vi "Laurel Meter Continuous Gather Tester.vi"(8 "Error In":errorcluster) -> (0 "Error Out":errorcluster)   [LabVIEW 2016]
uses:
  Trunk/Washer DOE/Type Definitions/DOE Test Fixture Hardware.ctl
  Trunk/Utility/Type Definitions/UTILITY Power Inputs Control.ctl
  IND560 Scale Monitor/Type Definitions/IND560 Configuration.ctl
  Trunk/Hybrid Water Heater/Type Definitions/HEWH Agilent Cluster.ctl
  Trunk/Utility/Type Definitions/UTILITY TC Coefficients.ctl
  Omega FMA-1600A Series Gas Flow Meter/Type Definitions/FMA1600A COM Ports.ctl
  Trunk/Washer DOE/Type Definitions/DOE Front Panel Meters.ctl
  Trunk/Utility/Type Definitions/UTILITY Power Data.ctl
  Trunk/Utility/Standby Power/Type Definitions/Standby Power Main Data.ctl
  Omega FMA-1600A Series Gas Flow Meter/Type Definitions/FMA1600A Gas Data.ctl
  Omega FMA-1600A Series Gas Flow Meter/Type Definitions/FMA1600A Gas Type.ctl
  Trunk/Range/Type Definitions/RANGE Meter Selector.ctl
  <vilib>/ptbypt/NI_PtbyPt.lvlib
panel:
  in  "Collect Meter (HOT,COLD,HOT COLD)":string
  in  "Laurel Communication Type":string
  in  "Rinse Button?":bool
  out "Loop Rate":dbl format="%0.2f"
  out "Header Data":string[][](array[string])
  in  "Measurments":T1 {"Power Measurements"."Voltage (V):Element 1 Avg" format="%.3g"; "Power Measurements"."Voltage (V):Element 2 Avg" format="%.3g"; "Power Measurements"."Max Watt Hours" format="%.3g"; "Power Measurements"."Power Factor:Element 2" format="%.3g"; "Power Measurements"."Power Factor:Element 1" format="%.3g"; "Power Measurements"."Apparent Power (VA):Element 2" format="%.3g"; "Power Measurements"."Apparent Power (VA):Element 1" format="%.3g"; "Power Measurements"."Frequency (Hz):Element 1" format="%.3g"; "Power Measurements"."Time:Element 1" format="%.3g"; "Power Measurements"."Voltage Crest Factor:Element 2" format="%.3g"; "Power Measurements"."Voltage Crest Factor:Element 1" format="%.3g"; "Power Measurements"."Voltage Harmonic Content (%):Element 2" format="%.3g"; "Power Measurements"."Voltage Harmonic Content (%):Element 1" format="%.3g"; "Power Measurements"."Current Crest Factor:Element 2" format="%.3g"; "Power Measurements"."Current Crest Factor:Element 1" format="%.3g"; "Power Measurements"."Voltage (V):Element 1" format="%.3g"; "Power Measurements"."Voltage (V):Element 2" format="%.3g"; "Power Measurements"."Watt Hours (Wh):Sigma" format="%.3g"; "Power Measurements"."Power (W):Sigma" format="%.3g"; "Power Measurements"."Current (A):Element 2" format="%.3g"; "Power Measurements"."Current (A):Element 1" format="%.3g"}
  in  "Fixture Hardware":T7={"Power "={"Yokogawa"={"WT210"={"Sample Rate (1: 0.25s)"=1, "A Range (12: 20A)"=11, "V Range (6: 600V)"=4, "Power VISA Yokogawa WT210"=""}, "WT500"={"Power VISA Yokogawa WT500"="", "V Range (8: 1000V)"=6, "I Range (7: 40A)"=7, "Update Rate (3: 500ms)"=2}, "WT310_2"={"Sample Rate (1: 0.25s)"=1, "A Range (12: 20A)"=11, "V Range (6: 600V)"=4, "Power VISA Yokogawa WT310_2"="WT310_2"}, "WT310_3"={"Sample Rate (1: 0.25s)"=1, "A Range (12: 20A)"=11, "V Range (6: 600V)"=4, "Power VISA Yokogawa WT310_3"="WT310_3"}}, "Aplus"={"Aplus IP Address"="192.168.1.101", "Remote Port"=502, "Instrument"="APLUS", "Instr Driver Revision"="1.03.0053"}, "Power Limits"={"Crest Factor"={"Upper Limit"=1.49, "Lower Limit"=1.34}, "Harmonic Content"={"Uthd"=2.0}, "Voltage"={"% Error"=2.0}, "Stability"={"<1 Watt "={"Wattage"=1.0, "Slope (mW/H)"=10.0}, ">1 Watt"={"1%Power/Hour"=1.0}}}, "Nominal Voltage"=120, "Time Limit (s)"=10800.0, "Power Variation Limit (%)"=50.0, "Power Supply"={"Chroma 61605"="CHROMA", "Use Chroma?"=FALSE}}, "Weight Scale"={"Com Options"={"IND560Scale VISA"="MW100", "IP Address"="", "Remote Port"=502, "Setra Scale VISA"="SETRA", "GSE 350"="GSE350"}, "Select Scale"=""}, "Flow Rates"={"Laurel Cold IP Address"="10.0.3.4", "Laurel Hot IP Address"="10.0.3.3", "Hot Water Laurel VISA"="LaurelMeter_Hot", "Cold Water Laurel VISA"="LaurelMeter_Cold", "Remote Port"=0, "Laurel Communication Type"="", "Meters To Collect (Hot Cold)"="", "HOT Laurel Reference"=refnum, "COLD Laurel Reference"=refnum}, "Analog Data"={"Agilent"={"Agilent 34972_1"="34972A_1", "Agilent 34972_2"="34972A_2", "Agilent 34972_3"="34972A_3", "Agilent 34972_4"="34972A_3", "Agilent 34972_5"="34972A_3", "Agilent 34972_6"="34972A_3", "Agilent Gain"=0.0, "TC Type (K,J,T)"="", "Instrument IDN?"="", "TC Channels-List"="", "Analog Channels-List"="", "Agilent Cluster Array"=[], "TC Channels-List 2"="", "Analog Channels-List 2"=""}, "Yokogawa"={"MW100"="MW100", "Intellifaucet"=FALSE}, "Select Analog"="", "TC Coefficients"={"TC Coefficients 1"=[], "TC Coefficients 2"=[], "TC Coefficients 3"=[], "TC Coefficients 4"=[], "TC Coefficients 5"=[], "TC Coefficients 6"=[], "TC Coefficients 7"=[]}, "NI Tasks (Dryer DOE)"=["TC Temps-Module 1", "TC Temps-Module 2", "TC Temps-Module 3", "TC Temps-Module 4", "TC Temps-Module 5", "Gas and Temp-Module 6", "AC_DC Events-Module 7"], "Laurel Analog"={"Laurel IP (Water Temp)"="", "Laurel IP (Pressure)"=""}}, "ITHX-Temp Humidity"={"IP Address 1"="", "Remote Port"=0, "IP Address 2"="", "IP Address 3"=""}, "Gas Meter COM Ports"={"Gas Meter 1"="COM3", "Gas Meter 2"="COM4", "Gas Meter 3"="COM5", "Gas Meter 4"="COM6", "Gas Meter 5"="COM7", "Gas Meter 6"="COM8"}, "Barometric Pressure"={"HEISE 901A"="HEISE", "Use Barometer?"=FALSE}} {"Power"."Yokogawa"."WT310_3"."V Range (6: 600V)" items=["Auto", "15V", "30V", "60V", "150V", "300V", "600V"]; "Power"."Yokogawa"."WT310_3"."A Range (12: 20A)" items=["Auto", "5mA", "10mA", "20mA", "50mA", "100mA", "200mA", "0.5A", "1A", "2A", "5A", "10A", "20A", "50mV", "100mV", "200mV", "2.5V", "5V", "10V"]; "Power"."Yokogawa"."WT310_3"."Sample Rate (1: 0.25s)" items=["0.1s", "0.25s", "0.5s", "1s", "2s", "5s"]; "Power"."Yokogawa"."WT310_2"."V Range (6: 600V)" items=["Auto", "15V", "30V", "60V", "150V", "300V", "600V"]; "Power"."Yokogawa"."WT310_2"."A Range (12: 20A)" items=["Auto", "5mA", "10mA", "20mA", "50mA", "100mA", "200mA", "0.5A", "1A", "2A", "5A", "10A", "20A", "50mV", "100mV", "200mV", "2.5V", "5V", "10V"]; "Power"."Yokogawa"."WT310_2"."Sample Rate (1: 0.25s)" items=["0.1s", "0.25s", "0.5s", "1s", "2s", "5s"]; "Power"."Yokogawa"."WT500"."Update Rate (3: 500ms)" items=["-", "100ms", "200ms", "500ms", "1s", "2s", "5s"]; "Power"."Yokogawa"."WT500"."I Range (7: 40A)" items=["AUTO", "500 mA", "1 A", "2 A", "5 A", "10 A", "20 A", "40 A", "S-AUTO", "50 mV", "100 mV", "200 mV", "500 mV", "1 V", "2 V", "5 V", "10 V", "250 mA", "500 mA", "1 A", "2.5 A", "5 A", "10 A", "20 A", "25 mV", "50 mV", "100 mV", "250 mV", "500 mV", "1 V", "2.5 V", "5 V"]; "Power"."Yokogawa"."WT500"."V Range (8: 1000V)" items=["AUTO", "15", "30", "60", "100", "150", "300", "600", "1000", "7.5", "15", "30", "50", "75", "150", "300", "500"]; "Power"."Yokogawa"."WT210"."V Range (6: 600V)" items=["Auto", "15V", "30V", "60V", "150V", "300V", "600V"]; "Power"."Yokogawa"."WT210"."A Range (12: 20A)" items=["Auto", "5mA", "10mA", "20mA", "50mA", "100mA", "200mA", "0.5A", "1A", "2A", "5A", "10A", "20A", "50mV", "100mV", "200mV", "2.5V", "5V", "10V"]; "Power"."Yokogawa"."WT210"."Sample Rate (1: 0.25s)" items=["0.1s", "0.25s", "0.5s", "1s", "2s", "5s"]}
  in  "stop":bool
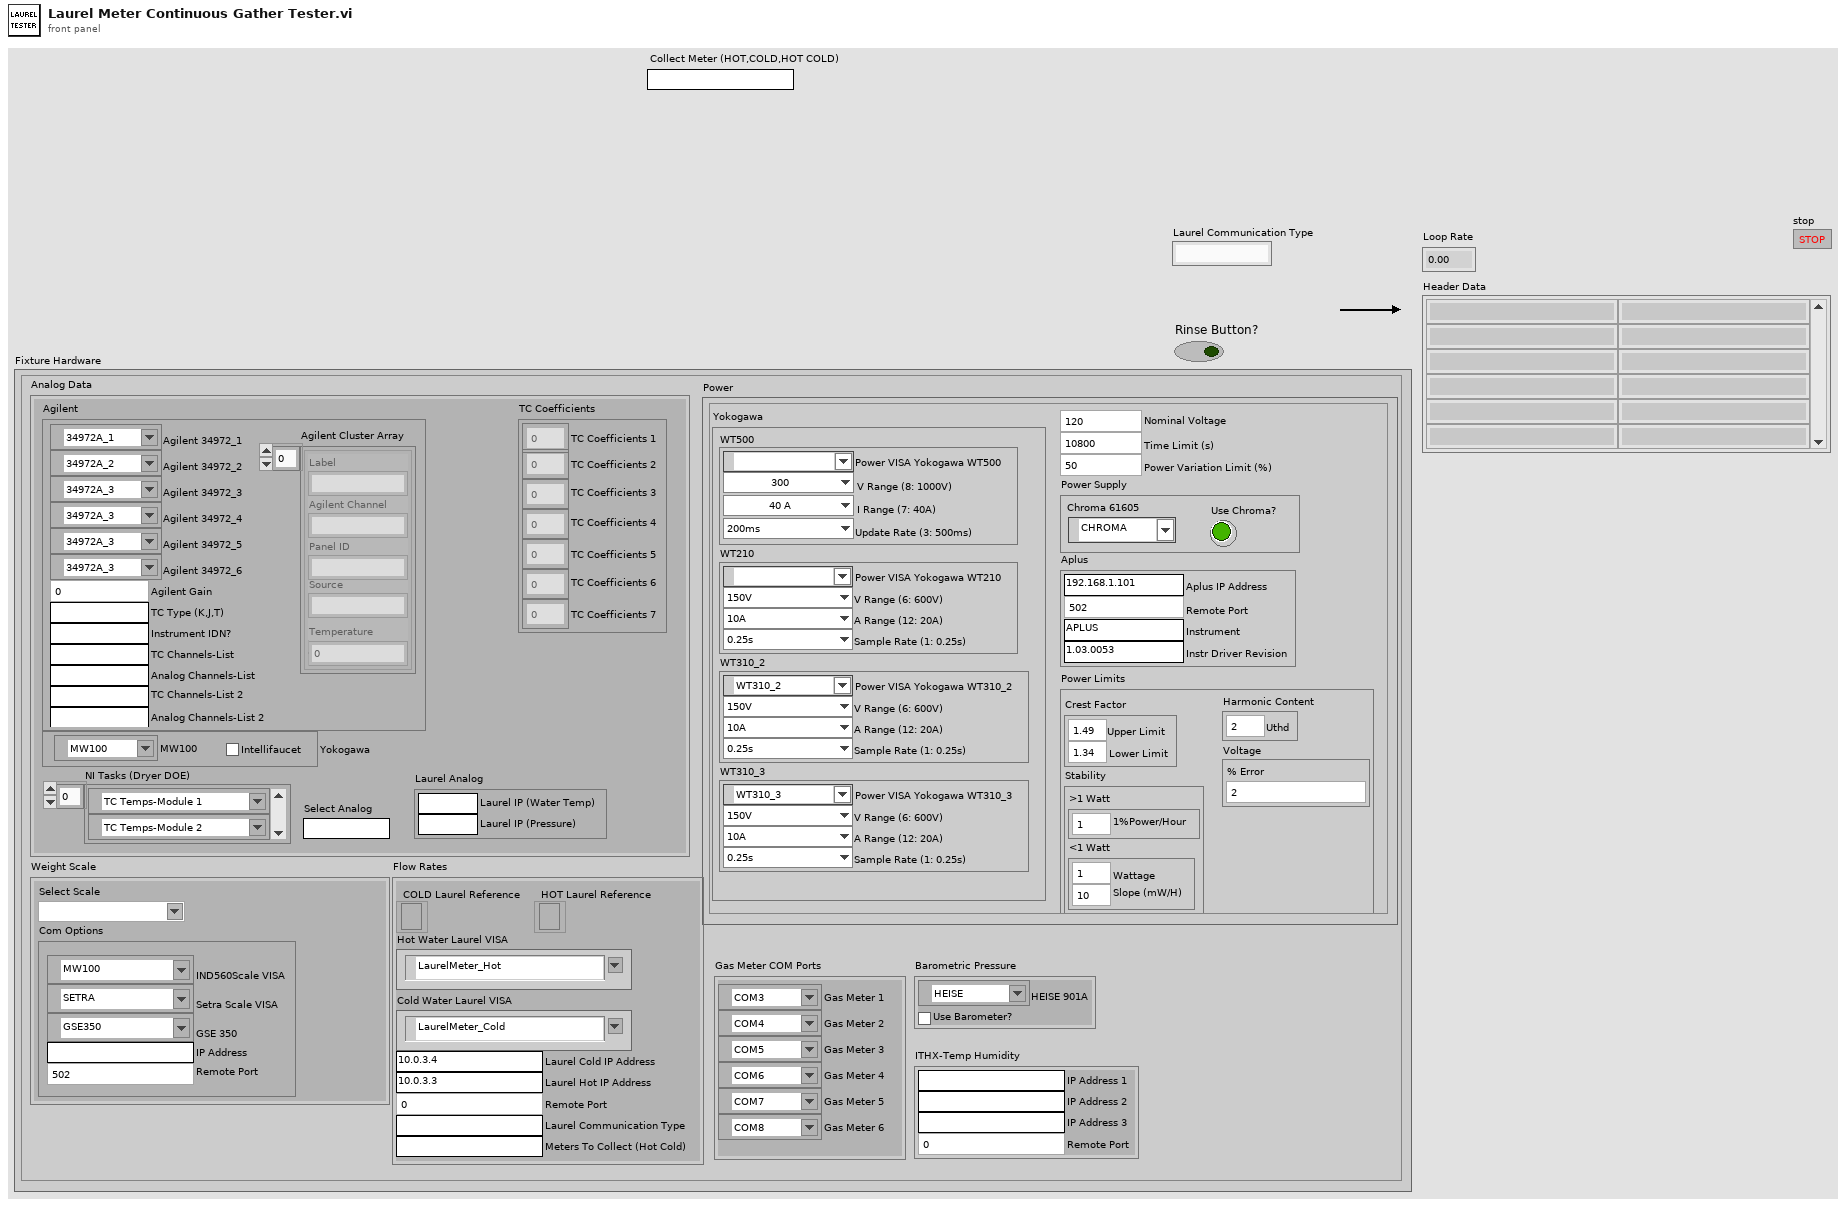
[diagram p1: front panel]
types:
  T1 = typedef "DOE Front Panel Meters.ctl" = cluster{"Power Measurements":T2, "Standby Power":T3, "Washer":cluster{"Washer String Data":string[][], "Analog Scale Weight (lbs)":dbl}, "Dishwasher":cluster{"Drain Solonoid Event":i32, "Pump Event":i32, "Water Valve Event":i32, "Heater Event":i32, "Motor Event":i32, "Turbidity Sensor":dbl, "Spare 2":dbl, "Spare 3":dbl, "Spare 4":dbl, "Spare 5":dbl, "Thermocouple 1":dbl, "Thermocouple 2":dbl, "Thermocouple 3":dbl, "Thermocouple 4":dbl, "Thermocouple 5":dbl, "Thermocouple 6":dbl, "Spare 1":dbl, "Dishwasher String Data":string[][]}, "Washer HCC":cluster{"Chan 101":dbl, "Chan 102":dbl, "Chan 103":dbl, "Chan 104":dbl, "Chan 105":dbl, "Chan 106":dbl, "Chan 107":dbl, "Chan 108":dbl, "Chan 109":dbl, "Chan 110":dbl, "Chan 111":dbl, "Chan 112":dbl, "Chan 113":dbl, "Chan 114":dbl, "Chan 115":dbl, "Chan 116":dbl, "Chan 117":dbl, "Chan 118":dbl, "Chan 119":dbl, "Chan 120":dbl, "Chan 201":dbl, "Chan 202":dbl, "Chan 203":dbl, "Chan 204":dbl, "Chan 205":dbl, "Chan 206":dbl, "Chan 207":dbl, "Chan 208":dbl, "Chan 209":dbl, "Chan 210":dbl, "Chan 211":dbl, "Chan 212":dbl, "Chan 213":dbl, "Chan 214":dbl, "Chan 215":dbl, "Chan 216":dbl, "Chan 217":dbl, "Chan 218":dbl, "Chan 219":dbl, "Chan 220":dbl, "Chan 301":dbl, "Chan 302":dbl, "Chan 303":dbl, "Chan 304":dbl, "Chan 305":dbl, "Chan 306":dbl, "Chan 307":dbl, "Chan 308":dbl, "Chan 309":dbl, "Chan 310":dbl, "Chan 311":dbl, "Chan 312":dbl, "Chan 313":dbl, "Chan 314":dbl, "Chan 315":dbl, "Chan 316":dbl, "Chan 317":dbl, "Chan 318":dbl, "Chan 319":dbl, "Chan 320":dbl}, "Barometric Pressure":cluster{"Barometric Pressure (in. Hg)":dbl}, "Ambient Conditions":cluster{"Ambient Temperature  1 (°F)":dbl, "Ambient Temperature 2 (°F)":dbl, "Ambient Temperature 3 (°F)":dbl, "Ambient Humidity 1 (%)":dbl, "Ambient Humidity 2 (%)":dbl, "Ambient Humidity 3 (%)":dbl, "Ambient Dewpoint  1 (°F)":dbl, "Ambient Dewpoint 2 (°F)":dbl, "Ambient Dewpoint 3 (°F)":dbl}, "Weight Scale":cluster{"Gross Weigth (lbs)":dbl, "Net Weight (lbs)":dbl, "Final Weight (lbs)":string}, "Water Measurements":cluster{"Hot Water Pressure (psi)":dbl, "Hot Water Pressure Avg (psi)":dbl, "Hot Water Temperature (°F)":dbl, "Cold Water Pressure (psi)":dbl, "Cold Water Pressure Avg (psi)":dbl, "Hot Water Temperature Avg (°F)":dbl, "Cold Water Temperature (°F)":dbl, "Cold Water Temperature Avg (°F)":dbl, "Hot Water Total (Gal)":dbl, "Hot Water Rate (GPM)":dbl, "Cold Water Total (Gal)":dbl, "Cold Water Rate (GPM)":dbl, "Cold Water Total During Wash (Gal)":dbl, "Hot Water Total During Wash (Gal)":dbl, "Rinse Cold (Gal)":dbl, "Rinse Hot (Gal)":dbl}, "Gas Data":T4}
  T2 = typedef "UTILITY Power Data.ctl" = cluster{"Current (A):Element 1":dbl, "Current (A):Element 2":dbl, "Power (W):Sigma":dbl, "Watt Hours (Wh):Sigma":dbl, "Voltage (V):Element 2":dbl, "Voltage (V):Element 1":dbl, "Current Crest Factor:Element 1":dbl, "Current Crest Factor:Element 2":dbl, "Voltage Harmonic Content (%):Element 1":dbl, "Voltage Harmonic Content (%):Element 2":dbl, "Voltage Crest Factor:Element 1":dbl, "Voltage Crest Factor:Element 2":dbl, "Time:Element 1":dbl, "Frequency (Hz):Element 1":dbl, "Apparent Power (VA):Element 1":dbl, "Apparent Power (VA):Element 2":dbl, "Power Factor:Element 1":dbl, "Power Factor:Element 2":dbl, "Max Watt Hours":dbl, "Voltage (V):Element 2 Avg":dbl, "Voltage (V):Element 1 Avg":dbl}
  T3 = typedef "Standby Power Main Data.ctl" = cluster{"Standby Power Spreadsheet":string[][], "Standby Power - Pia (Watts)":dbl, "Off Mode Power - Poff (Watts)":dbl, "Sia hr/yr":dbl, "Soff hr/yr":dbl, "Yearly Energy Etso kWh/yr":dbl, "Maximum Power (Watts)":dbl, "Power Variation (%)":dbl, "Slope (mW/hr)":dbl, "Final Harmonics-U1 (%)":string, "Final Harmonics-U2 (%)":string, "Energy (Wh)":dbl}
  T4 = typedef "FMA1600A Gas Data.ctl" = cluster{"Meter Type (Gas)":T5, "Meter ID":T6, "Heating Value (BTU/ft³)":dbl, "Ft³ / Hr (SCFH)":dbl, "15 Second Average (BTU/HR)":dbl, "30 Second Average (BTU/HR)":dbl, "SLPM (Mass Flow)":dbl, "LPM (Vol. Flow)":dbl, "Gas Temperature (°F)":dbl, "Gas Pressure (PSIA)":dbl, "Tot.Flow (Liters)":dbl}
  T5 = typedef "FMA1600A Gas Type.ctl" = string
  T6 = typedef "RANGE Meter Selector.ctl" = enum16{"Disabled", "Small", "Large"}
  T7 = typedef "DOE Test Fixture Hardware.ctl" = cluster{"Power ":T8, "Weight Scale":cluster{"Com Options":T9, "Select Scale":string}, "Flow Rates":cluster{"Laurel Cold IP Address":string, "Laurel Hot IP Address":string, "Hot Water Laurel VISA":refnum<visa-resource-name>, "Cold Water Laurel VISA":refnum<visa-resource-name>, "Remote Port":u16, "Laurel Communication Type":string, "Meters To Collect (Hot Cold)":string, "HOT Laurel Reference":refnum<k5>, "COLD Laurel Reference":refnum<k5>}, "Analog Data":cluster{"Agilent":cluster{"Agilent 34972_1":refnum<visa-resource-name>, "Agilent 34972_2":refnum<visa-resource-name>, "Agilent 34972_3":refnum<visa-resource-name>, "Agilent 34972_4":refnum<visa-resource-name>, "Agilent 34972_5":refnum<visa-resource-name>, "Agilent 34972_6":refnum<visa-resource-name>, "Agilent Gain":dbl, "TC Type (K,J,T)":string, "Instrument IDN?":string, "TC Channels-List":string, "Analog Channels-List":string, "Agilent Cluster Array":T10[], "TC Channels-List 2":string, "Analog Channels-List 2":string}, "Yokogawa":cluster{"MW100":refnum<visa-resource-name>, "Intellifaucet":bool}, "Select Analog":string, "TC Coefficients":T11, "NI Tasks (Dryer DOE)":refnum<k21>[], "Laurel Analog":cluster{"Laurel IP (Water Temp)":string, "Laurel IP (Pressure)":string}}, "ITHX-Temp Humidity":cluster{"IP Address 1":string, "Remote Port":u16, "IP Address 2":string, "IP Address 3":string}, "Gas Meter COM Ports":T12, "Barometric Pressure":cluster{"HEISE 901A":refnum<visa-resource-name>, "Use Barometer?":bool}}
  T8 = typedef "UTILITY Power Inputs Control.ctl" = cluster{"Yokogawa":cluster{"WT210":cluster{"Sample Rate (1: 0.25s)":i32, "A Range (12: 20A)":i32, "V Range (6: 600V)":i32, "Power VISA Yokogawa WT210":refnum<visa-resource-name>}, "WT500":cluster{"Power VISA Yokogawa WT500":refnum<visa-resource-name>, "V Range (8: 1000V)":i32, "I Range (7: 40A)":i32, "Update Rate (3: 500ms)":i32}, "WT310_2":cluster{"Sample Rate (1: 0.25s)":i32, "A Range (12: 20A)":i32, "V Range (6: 600V)":i32, "Power VISA Yokogawa WT310_2":refnum<visa-resource-name>}, "WT310_3":cluster{"Sample Rate (1: 0.25s)":i32, "A Range (12: 20A)":i32, "V Range (6: 600V)":i32, "Power VISA Yokogawa WT310_3":refnum<visa-resource-name>}}, "Aplus":cluster{"Aplus IP Address":string, "Remote Port":i32, "Instrument":string, "Instr Driver Revision":string}, "Power Limits":cluster{"Crest Factor":cluster{"Upper Limit":dbl, "Lower Limit":dbl}, "Harmonic Content":cluster{"Uthd":dbl}, "Voltage":cluster{"% Error":dbl}, "Stability":cluster{"<1 Watt ":cluster{"Wattage":dbl, "Slope (mW/H)":dbl}, ">1 Watt":cluster{"1%Power/Hour":dbl}}}, "Nominal Voltage":i32, "Time Limit (s)":dbl, "Power Variation Limit (%)":dbl, "Power Supply":cluster{"Chroma 61605":refnum<visa-resource-name>, "Use Chroma?":bool}}
  T9 = typedef "IND560 Configuration.ctl" = cluster{"IND560Scale VISA":refnum<visa-resource-name>, "IP Address":string, "Remote Port":u16, "Setra Scale VISA":refnum<visa-resource-name>, "GSE 350":refnum<visa-resource-name>}
  T10 = typedef "HEWH Agilent Cluster.ctl" = cluster{"Label":string, "Agilent Channel":string, "Panel ID":string, "Source":string, "Temperature":dbl}
  T11 = typedef "UTILITY TC Coefficients.ctl" = cluster{"TC Coefficients 1":dbl[], "TC Coefficients 2":dbl[], "TC Coefficients 3":dbl[], "TC Coefficients 4":dbl[], "TC Coefficients 5":dbl[], "TC Coefficients 6":dbl[], "TC Coefficients 7":dbl[]}
  T12 = typedef "FMA1600A COM Ports.ctl" = cluster{"Gas Meter 1":refnum<visa-resource-name>, "Gas Meter 2":refnum<visa-resource-name>, "Gas Meter 3":refnum<visa-resource-name>, "Gas Meter 4":refnum<visa-resource-name>, "Gas Meter 5":refnum<visa-resource-name>, "Gas Meter 6":refnum<visa-resource-name>}
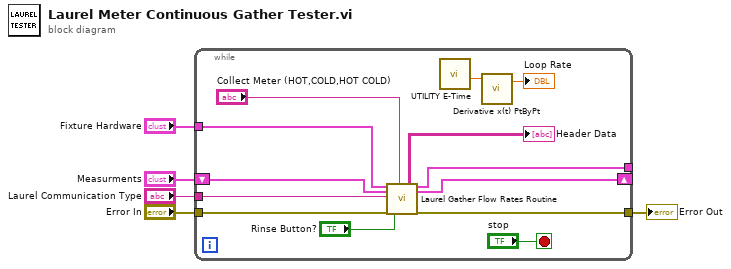
[diagram p0: block diagram]
diagram:
  n1 = while {
    tunnel: "Fixture Hardware" -> [w17]
    tunnel: [w14] -> _
    shift-right: [w13] -> _
    shift-left: "Measurments" -> [w16]
    tunnel: [w12] -> w3
    tunnel: "Error In" -> [w11]
    tunnel: "Laurel Communication Type" -> [w7]
    stop <- "stop" stop-if-true
    n2 = call "Laurel Gather Flow Rates Routine.vi"("Fixture Hardware"=w17, "Measurments"=w16, "Laurel Communication Type"=w7, "error in (no error)"=w11, "Rinse Button?"="Rinse Button?", "Collect Meter (HOT,COLD,HOT COLD)"="Collect Meter (HOT,COLD,HOT COLD)") -> ("Header Data"=→"Header Data":string[][], "Fixture Hardware Output"=w14:T7, "Measurments Output"=w13:T1, "error out"=w12:errorcluster)  [unwired: 9 in, 1 out]
    n3 = call "UTILITY E-Time.vi"() -> ("Elapsed Time (sec)"=w8:dbl)  [unwired: 9 in, 2 out]
    n4 = call <vilib>:"Derivative x(t) PtByPt.vi"("x"=w8) -> ("dx/dt"=→"Loop Rate":dbl)  [unwired: 3 in, 1 out]
  }
  "Error Out" <- w3
